vi "KalmanFilterLatencyComp_ApplyPastGlobalMeas_FuncGroup.vi"(6 "VisionCorrectExtra":variant, 7 "F_Func":T2, 8 "VisionCorrect_Func":refnum<vi>, 9 "H_FuncExtra":variant, 10 "H_Func":T2, 11 "F_FuncExtra":variant) -> (0 "Error":bool, 3 "KALMAN_FILTER_LATENCY_COMP_FUNC_GROUP":T1)   [LabVIEW 2019, in "Trajectory_Library.lvlib"]
doc: "Creates a new LINEAR SYSTEM data cluster with the specified values. \n\n\nInputs: \n - XXX -- XXX.\n\nOutputs:\n - XXX -- XXX."
uses:
  Trajectory_Library.lvlib
  CALLBACK_FUNC_TYPE.ctl
  KALMAN_FILTER_LATENCY_COMP_FUNC_GROUP.ctl
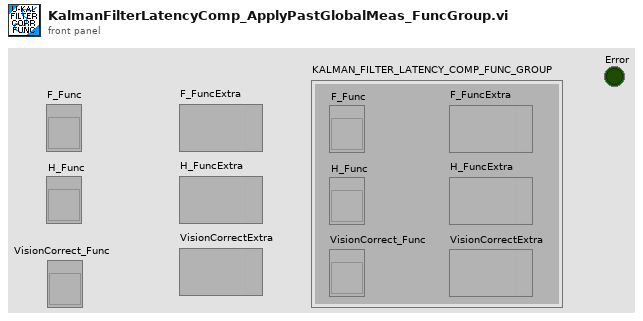
[diagram p1: front panel]
types:
  T1 = typedef "Trajectory_Library.lvlib/KALMAN_FILTER_LATENCY_COMP_FUNC_GROUP.ctl" = cluster{"F_Func":T2, "H_Func":T2, "F_FuncExtra":variant, "H_FuncExtra":variant, "VisionCorrectExtra":variant, "VisionCorrect_Func":refnum<vi>}
  T2 = typedef "Trajectory_Library.lvlib/CALLBACK_FUNC_TYPE.ctl" = refnum<vi>
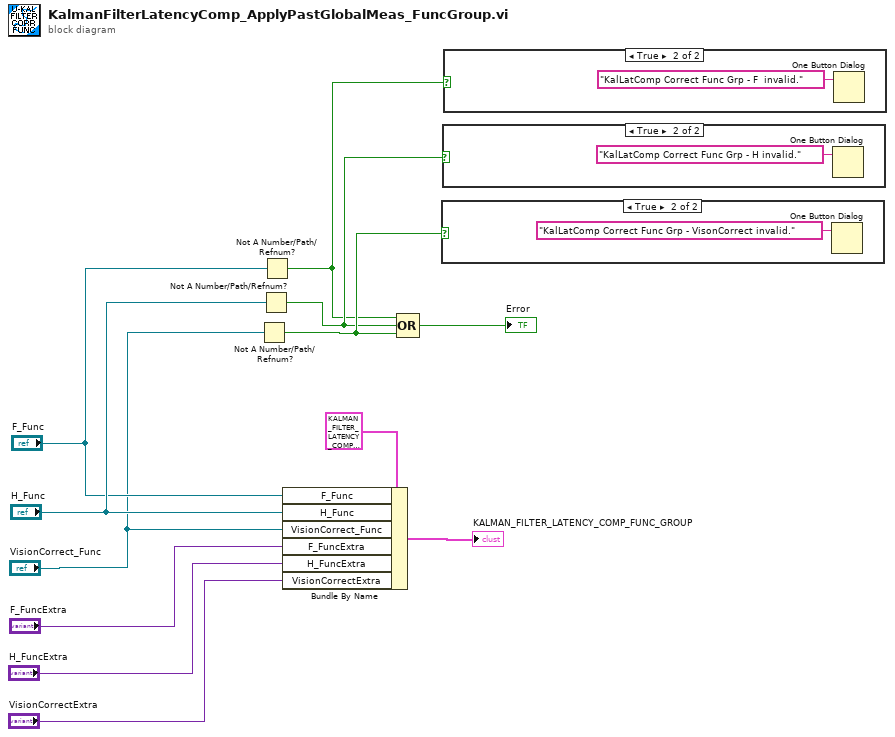
[diagram p0: block diagram]
diagram:
  n1 = Not A Number/Path/Refnum?(number/path/refnum="VisionCorrect_Func") -> (NaN/Path/Refnum?=w5:bool)
  n2 = Not A Number/Path/Refnum?(number/path/refnum="H_Func") -> (NaN/Path/Refnum?=w4:bool)
  n3 = Not A Number/Path/Refnum?(number/path/refnum="F_Func") -> (NaN/Path/Refnum?=w3:bool)
  n4 = Bundle By Name(cluster=T1 {"F_Func"=refnum, "H_Func"=refnum, "F_FuncExtra"=variant, "H_FuncExtra"=variant, "VisionCorrectExtra"=variant, "VisionCorrect_Func"=refnum} ("UNSCENTED_KALMAN_FILTER_FUNC_GROUP"), "F_Func"="F_Func", "H_Func"="H_Func", "VisionCorrect_Func"="VisionCorrect_Func", "F_FuncExtra"="F_FuncExtra", "H_FuncExtra"="H_FuncExtra", "VisionCorrectExtra"="VisionCorrectExtra") -> (→"KALMAN_FILTER_LATENCY_COMP_FUNC_GROUP":T1)
  n5 = Compound Arithmetic op=OR(w3, w4, w5) -> (→"Error":bool)
  n6 = case shown="True" w5 {
    frame False {
    }
    frame True {
      n7 = One Button Dialog(message="KalLatComp Correct Func Grp - VisonCorrect invalid.") -> ()  [unwired: 1 in, 1 out]
    }
  }
  n8 = case shown="True" w4 {
    frame False {
    }
    frame True {
      n9 = One Button Dialog(message="KalLatComp Correct Func Grp - H invalid.") -> ()  [unwired: 1 in, 1 out]
    }
  }
  n10 = case shown="True" w3 {
    frame False {
    }
    frame True {
      n11 = One Button Dialog(message="KalLatComp Correct Func Grp - F  invalid.") -> ()  [unwired: 1 in, 1 out]
    }
  }
